vi "sendCommandAndLog.vi"(8 "error in (no error)":errorcluster, 9 "woeking directory":path, 10 "command":string) -> (0 "error out":errorcluster, 2 "standard output":string)   [LabVIEW 2013, in "hgHandler.lvclass"]
uses:
  hgHandler/hgHandler.lvclass
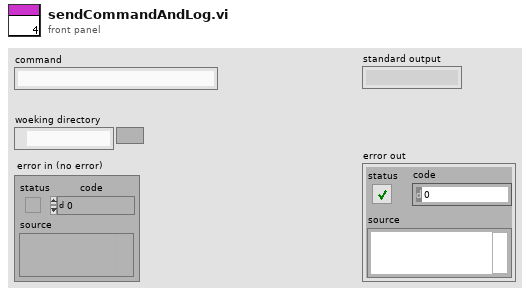
[diagram p1: front panel]
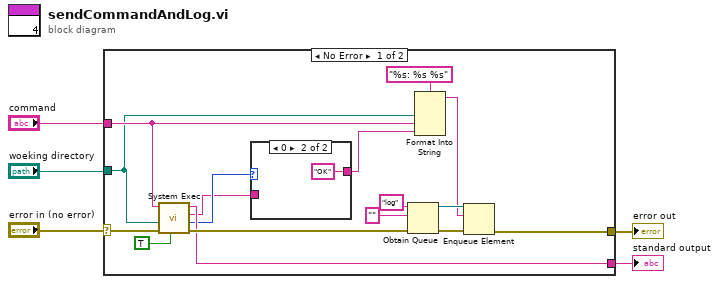
[diagram p0: block diagram]
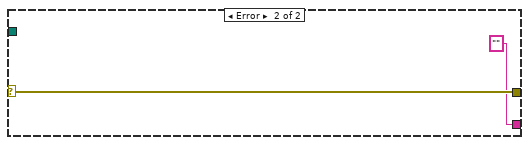
[diagram p3: hidden frame]
diagram:
  n1 = case shown="No Error" "error in (no error)" {
    selector: "error in (no error)" -> [w13 w25]
    tunnel: [w14 w25] -> w5
    tunnel: "command" -> [w8 _]
    tunnel: [w12 "" ("standard output")] -> w2
    tunnel: "woeking directory" -> [w6 _]
    frame No Error {
      n2 = call <vilib>:"System Exec.vi"("run minimized? (F)"=TRUE, "error in (no error)"=w13, "working directory"=w6, "command line"=w8) -> ("error out"=w20:errorcluster, "return code"=w11:i32, "standard error"=w10:string, "standard output"=w12:string)  [unwired: 4 in]
      n3 = case shown="0" w11 {
        tunnel: w10 -> [w22 _]
        tunnel: [w22 "OK" ("standard error")] -> w7
        frame Default {
        }
        frame 0 {
        }
      }
      n4 = Obtain Queue(name (unnamed)="log", element data type="", error in (no error)=w20) -> (queue out=w17:refnum<queue>, error out=w18:errorcluster)  [unwired: 2 in, 1 out]
      n5 = Format Into String(format string="%s: %s %s", w6, w8, w7) -> (resulting string=w16:string)  [unwired: 2 in, 1 out]
      n6 = Enqueue Element(queue=w17, element=w16, error in (no error)=w18) -> (error out=w14:errorcluster)  [unwired: 1 in, 2 out]
    }
    frame Error {
    }
  }
  "error out" <- w5
  "standard output" <- w2
